vi "String_Password.vi"(11 "String":string) -> (3 "Password":string)   [LabVIEW 2018]
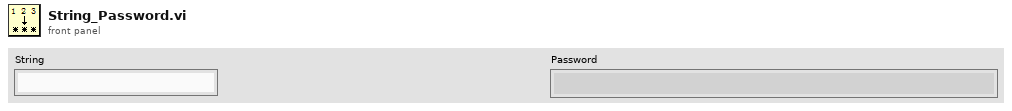
[diagram p1: front panel]
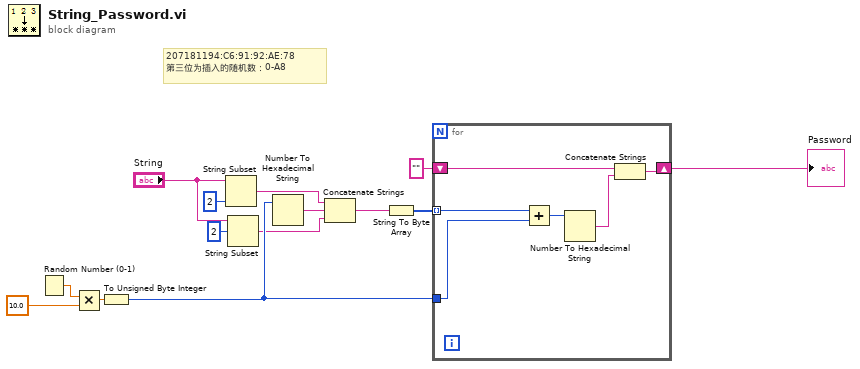
[diagram p0: block diagram]
diagram:
  # "207181194:C6:91:92:AE:78\n第三位为插入的随机数：0-A8"
  n1 = Random Number (0-1)() -> (number: 0 to 1=w13:dbl)
  n2 = Multiply(x=w13, y=10.0) -> (x*y=w11:dbl)
  n3 = To Unsigned Byte Integer(number=w11) -> (unsigned 8bit integer=w9:u8)
  n4 = String Subset(string="String", length (rest)=2 ("长度（剩余）")) -> (substring=w8:string)  [unwired: 1 in]
  n5 = String Subset(string="String", offset (0)=2 ("长度（剩余）")) -> (substring=w4:string)  [unwired: 1 in]
  n6 = Number To Hexadecimal String(2:w9) -> (0:w7:string)  [unwired: 1 in]
  n7 = Concatenate Strings(w8, w7, w4) -> (w3:string)
  n8 = String To Byte Array(string=w3) -> (unsigned byte array=w14:u8[])
  n9 = for {
    tunnel: w14 -> [w20] mode=indexing
    shift-right: [w17] -> w1
    shift-left: "" -> [w19]
    tunnel: w9 -> [w16]
    n10 = Add(x=w20, y=w16) -> (x+y=w15:u8)
    n11 = Number To Hexadecimal String(2:w15) -> (0:w18:string)  [unwired: 1 in]
    n12 = Concatenate Strings(w19, w18) -> (w17:string)
  }
  "Password" <- w1
